vi "Untitled 2.vi"() -> ()   [LabVIEW 2014]
uses:
  <vilib>/Instr/_visa.llb/VISA Configure Serial Port (Instr).vi
panel:
  out "Path #2 5":bool
  out "Path #2 4":bool
  out "Path #2 3":bool
  out "Path #2 2":bool
  in  "Calibration":bool
  out "Path #2":bool
  in  "VISA resource name":refnum<visa-resource-name>
  in  "error in (no error)":errorcluster
  out "error out":errorcluster
  out "path detector :":string
  in  "stop":bool
  in  "timeout (100 ms)":u32=10000
  in  "baud rate (115200)":u32=9600
  in  "data bits (8)":u16=8 min=5 max=8 step=1
  in  "parity (0:none)":enum16{"None", "Odd", "Even", "Mark", "Space"}(ring)
  in  "flow control (0:none)":u16(ring) items=["None", "XON/XOFF", "RTS/CTS", "XON/XOFF & RTS/CTS", "DTR/DSR", "XON/XOFF & DTR/DSR"]
  in  "stop bits (10: 1 bit)":u16(ring)=10 items=["1.0"=10, "1.5"=15, "2.0"=20]
  # "NODE 1"
  # "NODE 2"
  # "NODE 3"
  # "NODE 5"
  # "NODE 4"
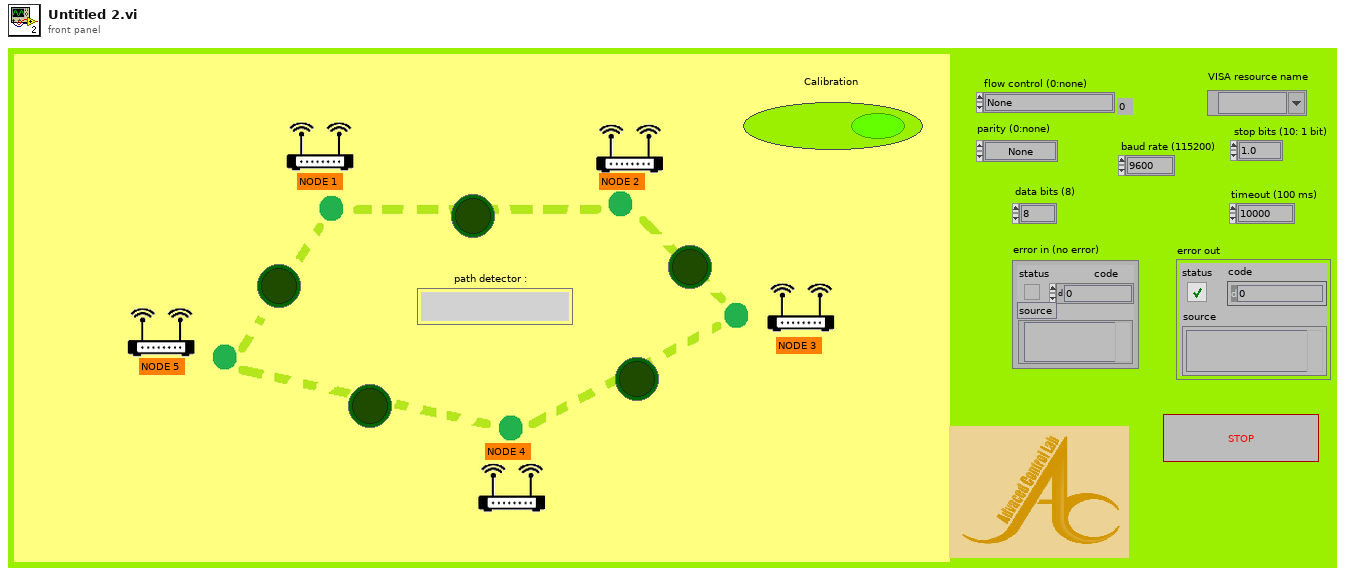
[diagram p1: front panel]
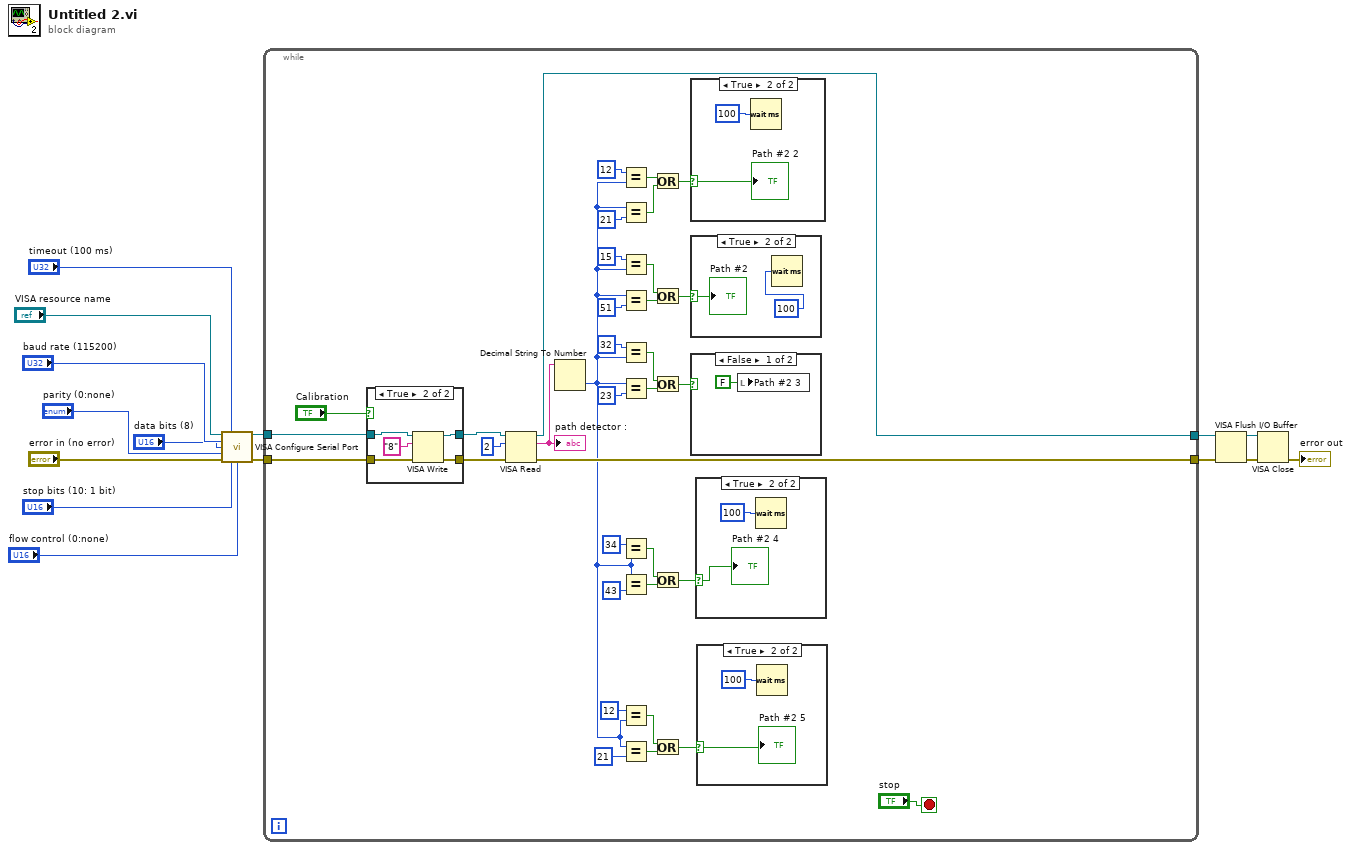
[diagram p0: block diagram]
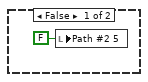
[diagram p2: hidden frame]
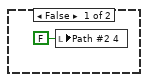
[diagram p3: hidden frame]
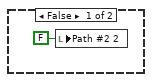
[diagram p5: hidden frame]
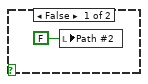
[diagram p6: hidden frame]
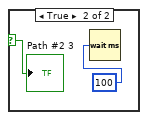
[diagram p7: hidden frame]
diagram:
  n1 = call-poly "VISA Configure Serial Port"("VISA resource name"="VISA resource name", "timeout (10sec)"="timeout (100 ms)", "baud rate (9600)"="baud rate (115200)", "data bits (8)"="data bits (8)", "parity (0:none)"="parity (0:none)", "error in (no error)"="error in (no error)", "stop bits (10: 1 bit)"="stop bits (10: 1 bit)", "flow control (0:none)"="flow control (0:none)") -> ("VISA resource name out"=w7:refnum<visa-resource-name>, "error out"=w8:errorcluster)  [unwired: 6 in]
  n2 = while {
    tunnel: w7 -> [w29]
    tunnel: w8 -> [w30]
    tunnel: [w49] -> w14
    tunnel: [w50] -> w12
    stop <- "stop" stop-if-true
    n3 = case shown="True" "Calibration" {
      tunnel: w30 -> [w59 w64]
      tunnel: [w59 w63] -> w27
      tunnel: [w58 w62] -> w28
      tunnel: w29 -> [w58 w60]
      frame False {
      }
      frame True {
        n4 = VISA Write(VISA resource name=w60, write buffer="8", error in (no error)=w64) -> (VISA resource name out=w62:refnum<visa-resource-name>, error out=w63:errorcluster)  [unwired: 1 out]
      }
    }
    n5 = VISA Read(VISA resource name=w28, byte count=2, error in (no error)=w27) -> (VISA resource name out=w50:refnum<visa-resource-name>, read buffer=w32:string, error out=w49:errorcluster)  [unwired: 1 out]
    "path detector :" <- w32
    n6 = Decimal String To Number(string=w32) -> (number=w16:i32)  [unwired: 2 in, 1 out]
    n7 = Equal?(x=12, y=w16) -> (x = y?=w34:bool)
    n8 = Equal?(x=w16, y=21) -> (x = y?=w35:bool)
    n9 = Equal?(x=15, y=w16) -> (x = y?=w39:bool)
    n10 = Equal?(x=w16, y=51) -> (x = y?=w41:bool)
    n11 = Equal?(x=32, y=w16) -> (x = y?=w44:bool)
    n12 = Equal?(x=w16, y=23) -> (x = y?=w42:bool)
    n13 = Equal?(x=34, y=w16) -> (x = y?=w25:bool)
    n14 = Equal?(x=w16, y=43) -> (x = y?=w23:bool)
    n15 = Equal?(x=12, y=w16) -> (x = y?=w21:bool)
    n16 = Equal?(x=w16, y=21) -> (x = y?=w19:bool)
    n17 = Or(x=w34, y=w35) -> (x .or. y?=w36:bool)
    n18 = Or(x=w39, y=w41) -> (x .or. y?=w46:bool)
    n19 = Or(x=w44, y=w42) -> (x .or. y?=w47:bool)
    n20 = Or(x=w25, y=w23) -> (x .or. y?=w17:bool)
    n21 = Or(x=w21, y=w19) -> (x .or. y?=w18:bool)
    n22 = case shown="True" w36 {
      selector: w36 -> [_ w66]
      frame False {
        n23 = local write "Path #2 2"(FALSE ("node #3")) -> ()
      }
      frame True {
        n24 = Wait (ms)(milliseconds to wait=u32 100) -> ()  [unwired: 1 out]
        "Path #2 2" <- w66
      }
    }
    n25 = case shown="True" w46 {
      selector: w46 -> [_ w70]
      frame False {
        n26 = local write "Path #2"(FALSE ("node #2")) -> ()
      }
      frame True {
        n27 = Wait (ms)(milliseconds to wait=u32 100 ("millisecond timer value")) -> ()  [unwired: 1 out]
        "Path #2" <- w70
      }
    }
    n28 = case shown="False" w47 {
      selector: w47 -> [_ w72]
      frame False {
        n29 = local write "Path #2 3"(FALSE ("node #1")) -> ()
      }
      frame True {
        n30 = Wait (ms)(milliseconds to wait=u32 100 ("millisecond timer value")) -> ()  [unwired: 1 out]
        "Path #2 3" <- w72
      }
    }
    n31 = case shown="True" w17 {
      selector: w17 -> [_ w56]
      frame False {
        n32 = local write "Path #2 4"(FALSE ("node #3")) -> ()
      }
      frame True {
        n33 = Wait (ms)(milliseconds to wait=u32 100) -> ()  [unwired: 1 out]
        "Path #2 4" <- w56
      }
    }
    n34 = case shown="True" w18 {
      selector: w18 -> [_ w53]
      frame False {
        n35 = local write "Path #2 5"(FALSE ("node #3")) -> ()
      }
      frame True {
        n36 = Wait (ms)(milliseconds to wait=u32 100) -> ()  [unwired: 1 out]
        "Path #2 5" <- w53
      }
    }
  }
  n37 = VISA Flush I/O Buffer(VISA resource name=w12, error in (no error)=w14) -> (VISA resource name out=w13:refnum<visa-resource-name>, error out=w15:errorcluster)  [unwired: 1 in]
  n38 = VISA Close(VISA resource name=w13, error in (no error)=w15) -> (error out=→"error out":errorcluster)
